vi "Global_HW_Data Out.vi"() -> ()   [LabVIEW 2017, in "TemplateSensor.lvlib"]
uses:
  TemplateSensor.lvlib
  Cluster_HW Status.ctl
panel:
  in  "HW_Status":T1
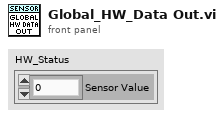
[diagram p1: front panel]
types:
  T1 = typedef "TemplateSensor.lvlib/Cluster_HW Status.ctl" = cluster{"Sensor Value":dbl}
diagram:
